vi "Predefined Demo.vi"(11 "Combo Box":string(combo)) -> (1 "Cancelled":bool, 3 "Value":string)   [LabVIEW 2020]
uses:
  <vilib>/Utility/miscctls.llb/LVComboBoxStrsAndValuesArrayTypeDef.ctl
  Dynamic Combobox/Dynamic Combobox/Options.ctl
  Dynamic Combobox/Predefined Values/Predefined Values.lvclass
  C:/dev/NI/Dynamic Combobox/Dynamic Combobox/Dynamic Values/Dynamic Values.lvclass
  Dynamic Combobox/Dynamic Combobox/Dynamic Combobox.lvclass
panel:
  out "error out":errorcluster
  out "Selected Value":string
  in  "Cancel Button":bool
  in  "OK Button":bool
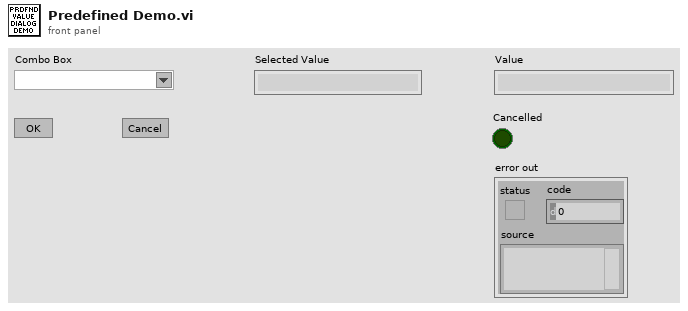
[diagram p1: front panel]
types:
  T1 = typedef "Dynamic Combobox.lvlib/Dynamic Combobox.lvclass/Options.ctl" = cluster{"Browse Entry":bool, "Refresh Entry":bool}
  T2 = typedef "LVComboBoxStrsAndValuesArrayTypeDef.ctl" = cluster{"String":string, "Value":string}[]
  T3 = typedef "Dynamic Combobox.lvlib/Dynamic Combobox.lvclass/Dynamic Combobox Events.ctl" = cluster{"Selection":refnum<user-event>, "Error":refnum<user-event>}
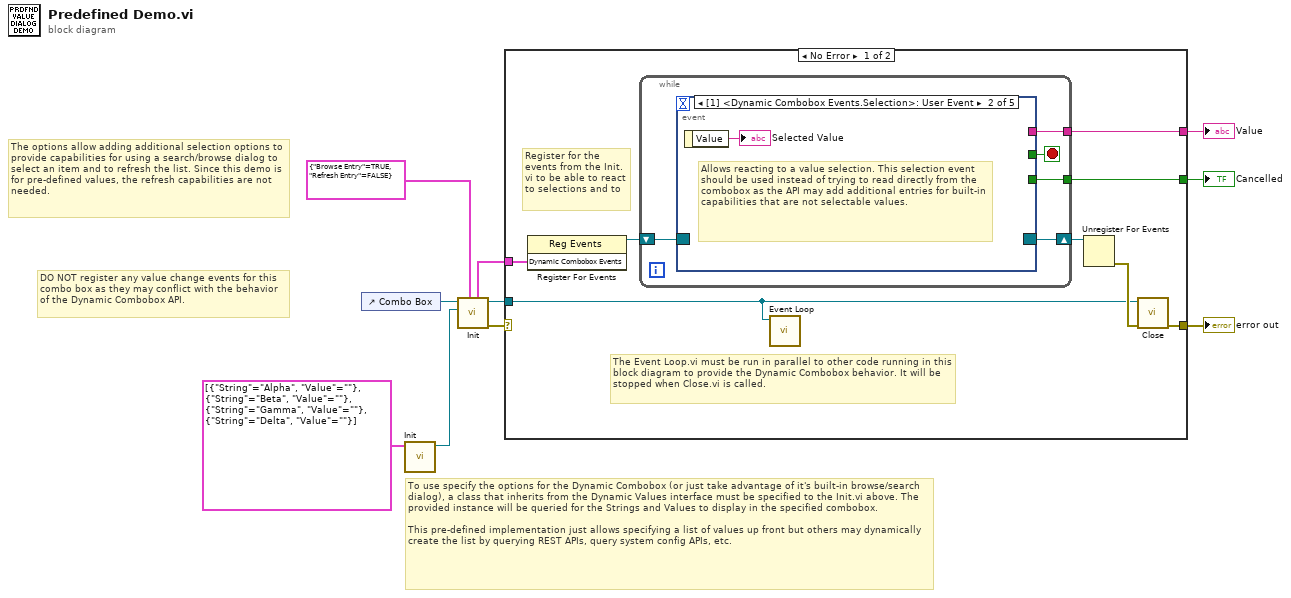
[diagram p0: block diagram]
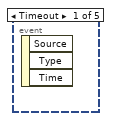
[diagram p2: hidden frame]
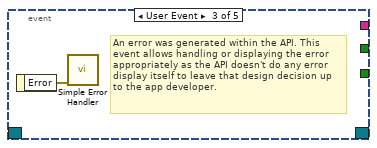
[diagram p3: hidden frame]
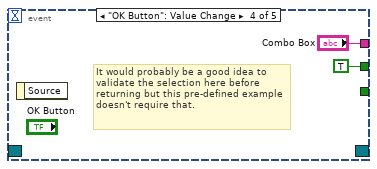
[diagram p4: hidden frame]
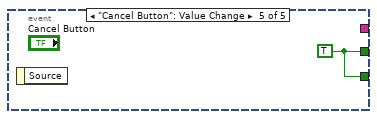
[diagram p5: hidden frame]
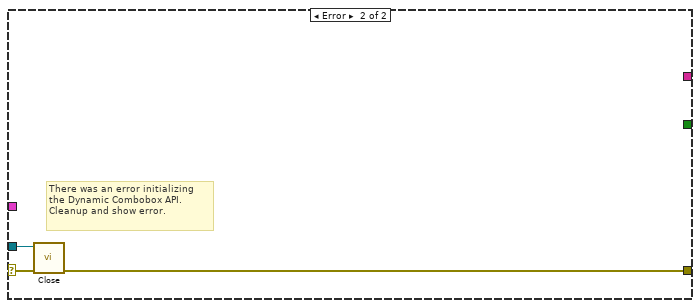
[diagram p6: hidden frame]
diagram:
  # "To use specify the options for the Dynamic Combobox (or just take advantage of it's built-in browse/search dialog), a class that inherits from the Dynamic Values interface must be specified to the Init.vi above. The provided instance will be queried for the Strings and Values to display in the specified combobox.\n\nThis pre-defined implementation just allows specifying a list of values up front but others may dynamically create the list by querying REST APIs, query system config APIs, etc."
  # "DO NOT register any value change events for this combo box as they may conflict with the behavior of the Dynamic Combobox API."
  # "The options allow adding additional selection options to provide capabilities for using a search/browse dialog to select an item and to refresh the list. Since this demo is for pre-defined values, the refresh capabilities are not needed."
  n1 = control-ref of="Combo Box"() -> (w10:refnum<vi>)
  n2 = call "Init.vi"("Strings And Values []"=T2 [{"String"="Alpha", "Value"=""}, {"String"="Beta", "Value"=""}, {"String"="Gamma", "Value"=""}, {"String"="Delta", "Value"=""}]) -> ("Predefined Values out"=w8:refnum<class "Predefined Values.lvclass">)  [unwired: 9 in, 1 out]
  n3 = call "Init.vi"("Options (None)"=T1 {"Browse Entry"=TRUE, "Refresh Entry"=FALSE} ("Options (Refresh First Open)"), "Dynamic Values"=w8, "Combobox"=w10) -> ("error out"=w2:errorcluster, "Dynamic Combobox out"=w4:refnum<class "Dynamic Combobox.lvclass">, "Dynamic Combobox Events"=w7:T3)  [unwired: 6 in]
  n4 = case shown="No Error" w2 {
    selector: w2 -> [_ w30]
    tunnel: w7 -> [w18 _]
    tunnel: [w15 _] -> w5
    tunnel: w4 -> [w11 w31]
    tunnel: [w14 _] -> w3
    tunnel: [w13 w29] -> w1
    frame No Error {
      # "The Event Loop.vi must be run in parallel to other code running in this block diagram to provide the Dynamic Combobox behavior. It will be stopped when Close.vi is called."
      # "Register for the events from the Init.vi to be able to react to selections and to"
      n5 = register-events(w18) -> (reference out=w17:refnum<event-registration>)  [unwired: 2 in, 1 out]
      n6 = while {
        shift-right: [w22] -> w16
        shift-left: w17 -> [w23]
        tunnel: [w20] -> w15
        tunnel: [w19] -> w14
        stop <- w21 stop-if-true
        n7 = event shown="[1] <Dynamic Combobox Events.Selection>: User Event" {
          selector: w23 -> [_ _ _ _ _]
          dyn-events: [_ _ _ _ _] -> w22
          timeout: _ -> [_ _ _ _ _]
          tunnel: [_ _ _ TRUE ("Valid") w28] -> w21
          tunnel: [_ _ _ "Combo Box" _] -> w20
          tunnel: [_ _ _ _ w28] -> w19
          event Timeout {
            n8 = event-data() -> ()  [unwired: 1 in, 3 out]
          }
          event User Event {
            # "Allows reacting to a value selection. This selection event should be used instead of trying to read directly from the combobox as the API may add additional entries for built-in capabilities that are not selectable values."
            n9 = event-data() -> ("Value"=→"Selected Value":string)  [unwired: 1 in]
          }
          event User Event {
            # "An error was generated within the API. This event allows handling or displaying the error appropriately as the API doesn't do any error display itself to leave that design decision up to the app developer."
            n10 = event-data() -> ("Error"=w25:errorcluster)  [unwired: 1 in]
            n11 = call <vilib>:"Simple Error Handler.vi"("error in (no error)"=w25) -> ()  [unwired: 4 in, 5 out]
          }
          event "OK Button": Value Change {
            # "It would probably be a good idea to validate the selection here before returning but this pre-defined example doesn't require that."
            n12 = event-data() -> ()  [unwired: 1 in, 1 out]
          }
          event "Cancel Button": Value Change {
            w28 = TRUE ("Valid")
            n13 = event-data() -> ()  [unwired: 1 in, 1 out]
          }
        }
      }
      n14 = call "Event Loop.vi"("Dynamic Combobox in"=w11) -> ()  [unwired: 10 in, 1 out]
      n15 = Unregister For Events(event registration refnum=w16) -> (error out=w12:errorcluster)  [unwired: 1 in]
      n16 = call "Close.vi"("error in (no error)"=w12, "Dynamic Combobox in"=w11) -> ("error out"=w13:errorcluster)  [unwired: 9 in]
    }
    frame Error {
      # "There was an error initializing the Dynamic Combobox API. Cleanup and show error."
      n17 = call "Close.vi"("error in (no error)"=w30, "Dynamic Combobox in"=w31) -> ("error out"=w29:errorcluster)  [unwired: 9 in]
    }
  }
  "Cancelled" <- w3
  "Value" <- w5
  "error out" <- w1
